vi "Put (U32 Array).vi"(6 "timestamp in":timestamp, 7 "PV name":string, 8 "error in (no error)":errorcluster, 9 "timeout":dbl[unit]=1.0, 10 "value in":u32[](array[numeric]), 11 "Client in":refnum<class "Client.lvclass">) -> (0 "error out":errorcluster, 1 "timed out?":bool, 2 "value out":u32[](array[numeric]), 3 "Client out":refnum<class "Client.lvclass">, 4 "timestamp out":timestamp)   [LabVIEW 2020, in "PV Access.lvlib" / "PVA Client.lvlib" / "Client.lvclass"]
uses:
  Client.lvclass
  PV Data/PV Data/PV Data.lvclass
  09055bfe-3840-473e-8f73-dd572ee5ee6f.vi
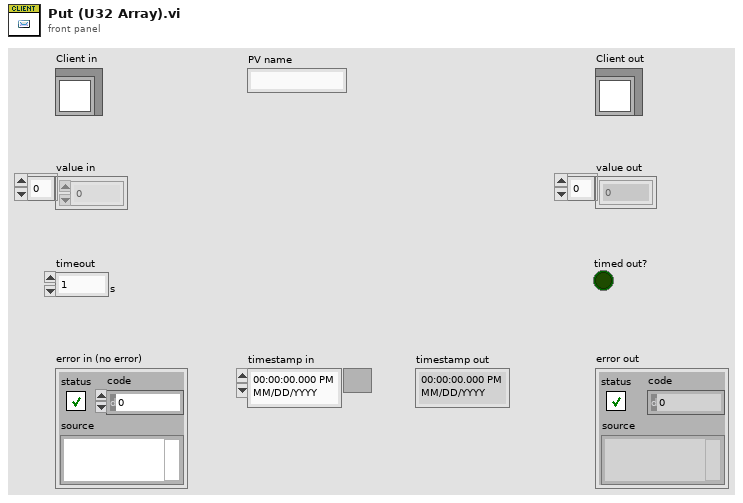
[diagram p1: front panel]
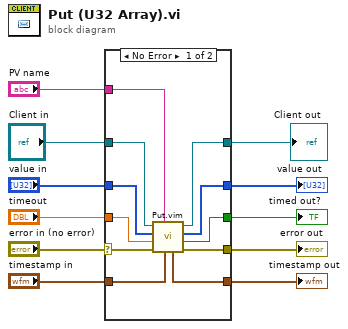
[diagram p0: block diagram]
diagram:
  n1 = case shown="No Error" "error in (no error)" {
    selector: "error in (no error)" -> [w15 w26]
    tunnel: [w14 w26] -> w10
    tunnel: [w16 w25] -> w8
    tunnel: "Client in" -> [w17 w25]
    tunnel: "value in" -> [w22 w24]
    tunnel: [w21 w24] -> w6
    tunnel: "timeout" -> [w20 _]
    tunnel: [w19 _] -> w4
    tunnel: "PV name" -> [w18 _]
    tunnel: "timestamp in" -> [w13 w23]
    tunnel: [w12 w23] -> w1
    frame No Error {
      n2 = call "Put.vim"("timestamp"=w13, "PV name"=w18, "error in"=w15, "timeout"=w20, "value in"=w22, "Client in"=w17) -> ("error out"=w14:errorcluster, "timed out?"=w19:bool, "value out"=w21:u32[], "Client out"=w16:refnum<class "Client.lvclass">, "timestamp out"=w12:timestamp)  [unwired: 1 in]
    }
    frame Error {
    }
  }
  "error out" <- w10
  "Client out" <- w8
  "value out" <- w6
  "timed out?" <- w4
  "timestamp out" <- w1
